vi "Test.vi"(0 "location":T3(ring), 1 "saved x":i32, 2 "saved y":i32, 3 "user_x":i32, 4 "user_y":i32, 5 "error in (no error)":errorcluster, 8 "IN?":bool) -> (14 "Nearest Detector":string, 16 "Status":T1, 17 "Distance from user (meters)":sgl, 19 "error out":errorcluster)   [LabVIEW 2020]
uses:
  Controls/Book_Status.ctl
  <vilib>/vision/NI_Vision_Development_Module.lvlib
panel:
  out "Image Out":T2(plugin-control)
  out "generated coordinates":cluster{"X":sgl, "Y":sgl}
  # "Initial status from OPAC DB:"
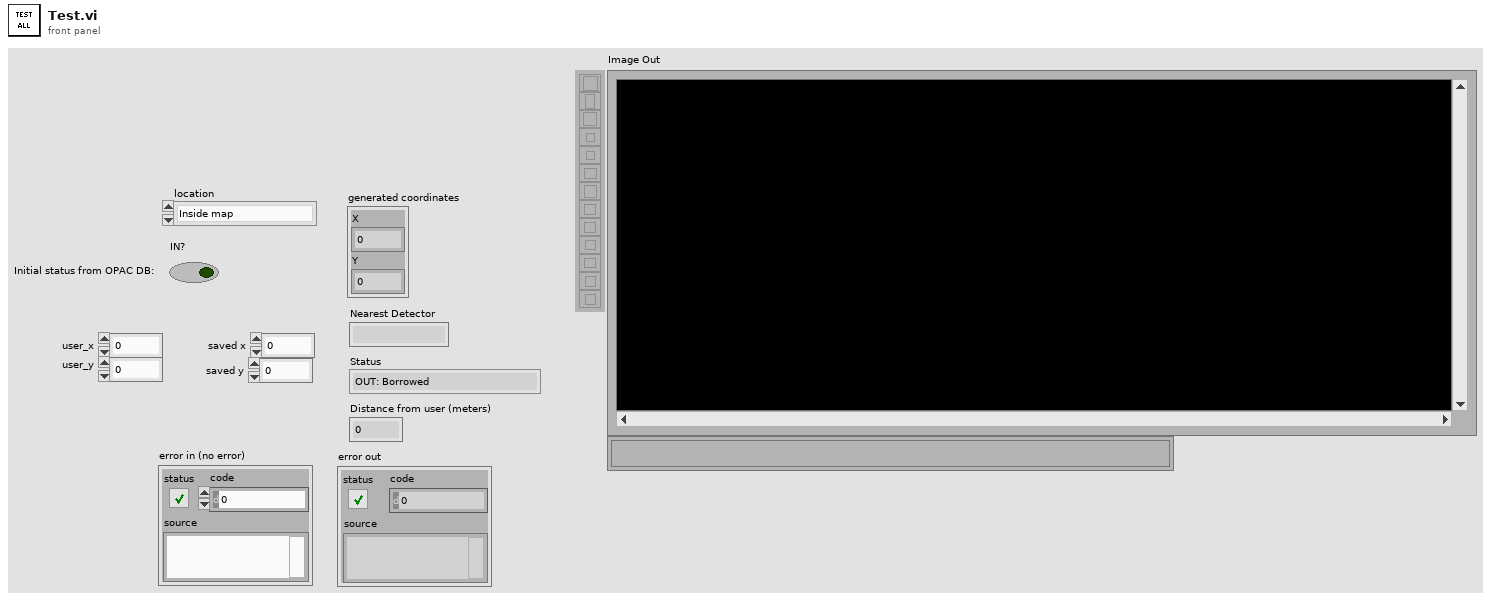
[diagram p1: front panel]
types:
  T1 = typedef "Book_Status.ctl" = enum16{"OUT: Borrowed", "OUT: In Segregation Machine", "IN: Currently In Use", "IN: Available", "IN: Misplaced", "IN: Location not found"}
  T2 = typedef "IMAQ Image.ctl" = refnum<image>
  T3 = enum16{"Inside map", "Anywhere", "Near saved location"}
  T4 = typedef "Image_Cluster.ctl" = cluster{"Detector_info":cluster{"No. of detectors":dbl, "Detector_Array":string[][], "Detector_Array_Numeric":dbl[][]}, "Corner_info":cluster{"Corner_Array":dbl[][]}, "ROI":cluster{"Corners":cluster{"Global Rectangle":i32[], "Contours":cluster{"ID":enum32{"External", "Internal"}, "Type":u32, "Coordinates":i32[]}[]}[], "Detectors":cluster{"Global Rectangle":i32[], "Contours":cluster{"ID":enum32{"External", "Internal"}, "Type":u32, "Coordinates":i32[]}[]}[]}, "Shape_Detect":cluster{"Match_score":dbl, "Curve Parameters":T5, "Match Options":T6, "Circle Descriptor":cluster{"Min Radius":dbl, "Max Radius":dbl}}, "Path":cluster{"Config":path, "Map":path}, "Map":cluster{"X_resolution":i32, "Y_resolution":i32, "Image":T2, "Image_colored":T2}, "Conversion_factor":dbl}
  T5 = typedef "IMAQ Curve Parameters.ctl" = cluster{"Extraction Mode":u32, "Edge Threshold":i32, "Edge Filter Size":u32, "Min Length":i32, "Row Search Step Size":i32, "Col Search Step Size":i32, "Max Endpoint Gap":i32, "Closed":bool, "Subpixel":bool}
  T6 = typedef "ShapeDetectionMatchOptions.ctl" = cluster{"Rotation":bool, "Scale":bool, "Occlusion":bool, "Range Settings":T7[]}
  T7 = typedef "IMAQ Match Range Setting.ctl" = cluster{"Match Constraints":u32, "Min":dbl, "Max":dbl}
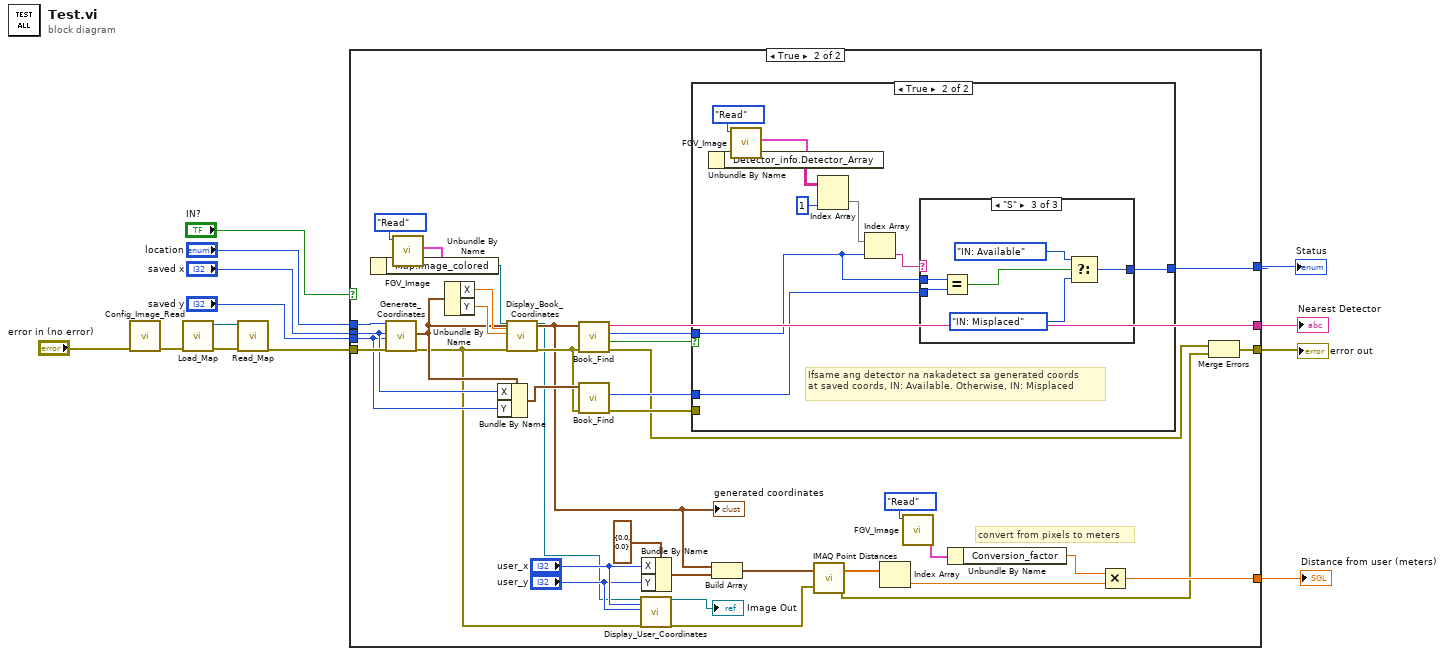
[diagram p0: block diagram]
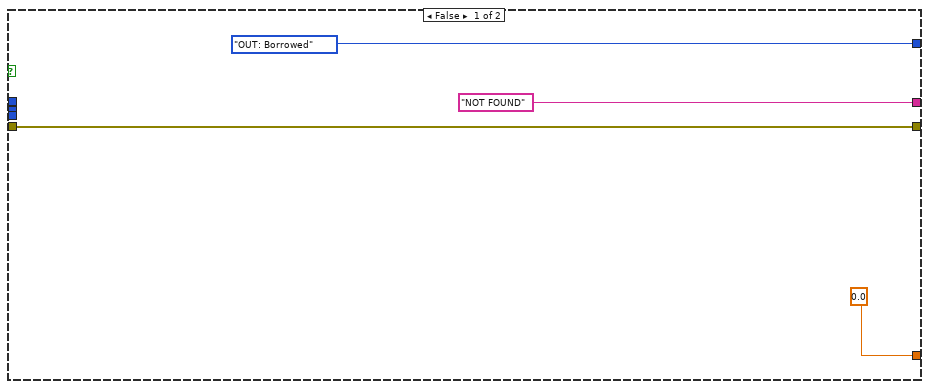
[diagram p2: hidden frame]
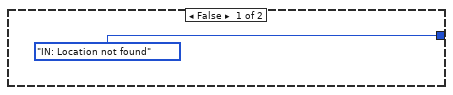
[diagram p3: hidden frame]
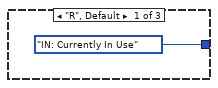
[diagram p4: hidden frame]
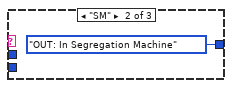
[diagram p5: hidden frame]
diagram:
  n1 = call "Config_Image_Read.vi"("error in (no error)"="error in (no error)") -> ("error out"=w13:errorcluster)  [unwired: 10 in]
  n2 = call "Load_Map.vi"("error in (no error)"=w13) -> ("error out"=w11:errorcluster, "Image Out"=w1:T2)  [unwired: 7 in, 1 out]
  n3 = call "Read_Map.vi"("error_in"=w11, "Image In"=w1) -> ("error out"=w10:errorcluster)  [unwired: 9 in]
  n4 = case shown="True" "IN?" {
    tunnel: w10 -> [w16 w53]
    tunnel: "location" -> [_ w52]
    tunnel: "saved x" -> [_ w44]
    tunnel: "saved y" -> [_ w43]
    tunnel: [w16 w32] -> w6
    tunnel: ["NOT FOUND" ("Nearest Detector") w49] -> w5
    tunnel: [Book_Status."OUT: Borrowed" ("Status") w47] -> w3
    tunnel: [sgl 0.0 w34] -> w2
    frame False {
    }
    frame True {
      # "convert from pixels to meters"
      n5 = call "Generate_Coordinates.vi"("location"=w52, "saved x"=w44, "saved y"=w43, "error in (no error)"=w53) -> ("generated coordinates"=w37:cluster{"X":sgl, "Y":sgl}, "error IO"=w26:errorcluster)  [unwired: 14 in]
      "generated coordinates" <- w37
      n6 = call "FGV_Image.vi"("Action"=enum16{"Read", "Write", ""}."Read") -> ("Image_Cluster_out"=w19:T4)  [unwired: 10 in]
      n7 = Unbundle By Name(w19) -> ("Map.Image_colored"=w18:T2)
      n8 = Unbundle By Name(w37) -> ("X"=w51:sgl, "Y"=w50:sgl)
      n9 = Bundle By Name(cluster=w37, "X"=w44, "Y"=w43) -> (w45:cluster{"X":sgl, "Y":sgl})
      n10 = call "Display_Book_Coordinates.vi"("Image In"=w18, "x"=w51, "y"=w50, "error in (no error)"=w26) -> ("Image Out"=w21:T2, "error out"=w42:errorcluster)  [unwired: 14 in]
      n11 = call "Book_Find.vi"("error in (no error)"=w42, "generated coordinates"=w37) -> ("error out"=w31:errorcluster, "Found?"=w48:bool, "Detector Index"=w46:i32, "Nearest Detector"=w49:string)  [unwired: 6 in]
      n12 = call "Book_Find.vi"("error in (no error)"=w42, "generated coordinates"=w45) -> ("error out"=w41:errorcluster, "Detector Index"=w40:i32)  [unwired: 6 in, 2 out]
      n13 = call "Display_User_Coordinates.vi"("Image In"=w21, "x"="user_x", "y"="user_y", "error in (no error)"=w26) -> ("Image Out"=→"Image Out":T2, "error out"=w25:errorcluster)  [unwired: 14 in]
      n14 = Bundle By Name(cluster=cluster{"X":sgl, "Y":sgl} {"X"=0.0, "Y"=0.0}, "X"="user_x", "Y"="user_y") -> (w39:cluster{"X":sgl, "Y":sgl})
      n15 = case shown="True" w48 {
        tunnel: [Book_Status."IN: Location not found" ("Status") w57] -> w47
        tunnel: w46 -> [_ w55]
        tunnel: w41 -> [_ _]
        tunnel: w40 -> [_ w56]
        frame False {
        }
        frame True {
          # "Ifsame ang detector na nakadetect sa generated coords\nat saved coords, IN: Available. Otherwise, IN: Misplaced"
          n16 = call "FGV_Image.vi"("Action"=enum16{"Read", "Write", ""}."Read") -> ("Image_Cluster_out"=w63:T4)  [unwired: 10 in]
          n17 = Unbundle By Name(w63) -> ("Detector_info.Detector_Array"=w61:string[][])
          n18 = Index Array(array=w61, index (col)=1 ("disabled index (col)")) -> (element=w59:string[])  [unwired: 1 in]
          n19 = Index Array(array=w59, index=w55) -> (element=w58:string)
          n20 = case shown="\"S\"" w58 {
            tunnel: [Book_Status."IN: Currently In Use" ("Status") Book_Status."OUT: In Segregation Machine" ("Status") w66] -> w57
            tunnel: w56 -> [_ _ w70]
            tunnel: w55 -> [_ _ w71]
            frame "R", Default {
            }
            frame "SM" {
            }
            frame "S" {
              n21 = Equal?(x=w71, y=w70) -> (x = y?=w67:bool)
              n22 = Select(t=Book_Status."IN: Available" ("Status"), s=w67, f=Book_Status."IN: Misplaced" ("Status")) -> (s? t:f=w66:T1)
            }
          }
        }
      }
      n23 = Build Array(w37, w39) -> (w36:cluster{"X":sgl, "Y":sgl}[])
      n24 = call "IMAQ Point Distances"("Points"=w36, "error in (no error)"=w25) -> ("Distances"=w35:sgl[], "error out"=w30:errorcluster)  [unwired: 3 in]
      n25 = Index Array(array=w35) -> (element=w33:sgl)  [unwired: 1 in]
      n26 = call "FGV_Image.vi"("Action"=enum16{"Read", "Write", ""}."Read") -> ("Image_Cluster_out"=w28:T4)  [unwired: 10 in]
      n27 = Unbundle By Name(w28) -> ("Conversion_factor"=w27:dbl)
      n28 = Multiply(x=w27, y=w33) -> (x*y=w34:dbl)
      n29 = Merge Errors(w31, w30) -> (w32:errorcluster)
    }
  }
  "error out" <- w6
  "Status" <- w3
  "Nearest Detector" <- w5
  "Distance from user (meters)" <- w2
